vi "Команда обмена 85 (обновление парам. мишени с  id ) (SubVI).vi"(2 "id мишени":u16, 4 "Выстрелов осталось":u16, 7 "error in":errorcluster, 9 "TCP connection ID":refnum<k5>, 11 "Выстрелов до перемотки":u16, 13 "До перемотки осталось":u16) -> (27 "error out":errorcluster)   [LabVIEW 2013]
doc: "Команда 85 - инициировать запрос на обновление параметров мишени с переданным id"
panel:
  out "string":string
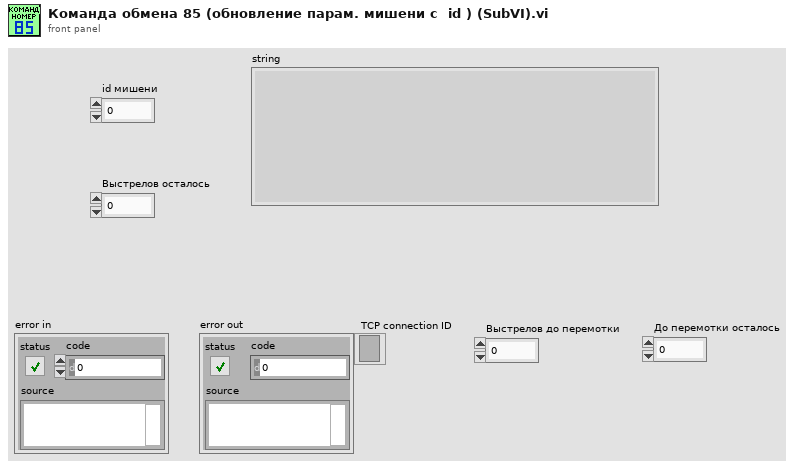
[diagram p1: front panel]
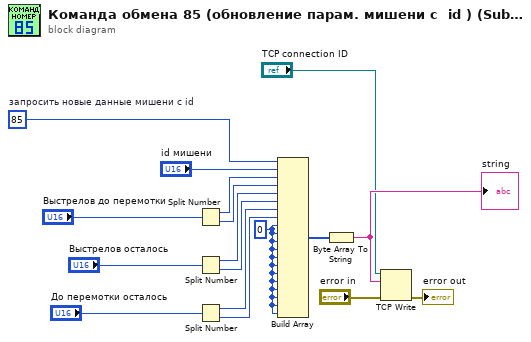
[diagram p0: block diagram]
diagram:
  w16 = u16 0 ("element")
  w2 = u8 85  # запросить новые данные мишени с id
  n1 = Split Number(x="Выстрелов до перемотки") -> (hi(x)=w8:u8, lo(x)=w9:u8)
  n2 = Split Number(x="Выстрелов осталось") -> (hi(x)=w14:u8, lo(x)=w15:u8)
  n3 = Split Number(x="До перемотки осталось") -> (hi(x)=w11:u8, lo(x)=w12:u8)
  n4 = Build Array(w2, "id мишени", w8, w9, w14, w15, w11, w12, w16, w16, w16, w16, w16, w16, w16, w16, w16, w16, w16, w16) -> (w3:u16[])
  n5 = Byte Array To String(unsigned byte array=w3) -> (string=w5:string)
  "string" <- w5
  n6 = TCP Write(connection ID="TCP connection ID", data in=w5, error in (no error)="error in") -> (error out=→"error out":errorcluster)  [unwired: 1 in, 2 out]
